vi "_GetKeys.vi"(8 "error in (no error)":errorcluster, 11 "EventBag in":refnum<class "EventBag.lvclass">) -> (0 "error out":errorcluster, 2 "Keys":refnum<class "EventToken.lvclass">[](array[class]), 3 "EventBag out":refnum<class "EventBag.lvclass">)   [LabVIEW 2009, in "EventManagerLibrary.lvlib" / "EventBag.lvclass"]
uses:
  EventBag.lvclass
  EventToken/EventToken.lvclass
  EventBag.lvclass/EventBag.ctl
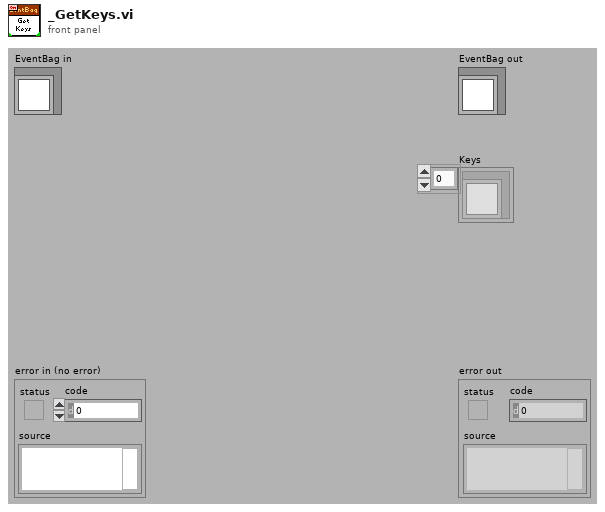
[diagram p1: front panel]
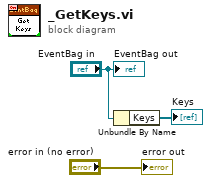
[diagram p0: block diagram]
diagram:
  n1 = Unbundle By Name("EventBag in") -> ("Keys"=→"Keys":refnum<class "EventToken.lvclass">[])
  "error out" <- "error in (no error)"
  "EventBag out" <- "EventBag in"
